vi "f-c_temperature.vi"(10 "Fahrenheit":dbl) -> (2 "Celsius":dbl)   [LabVIEW 2023]
panel:
  out "Thermometer":dbl(slide) scale=0.0..100.0
  out "Numeric 2":dbl
  in  "Numeric":dbl
  out "?":dbl(slide) scale=0.0..100.0
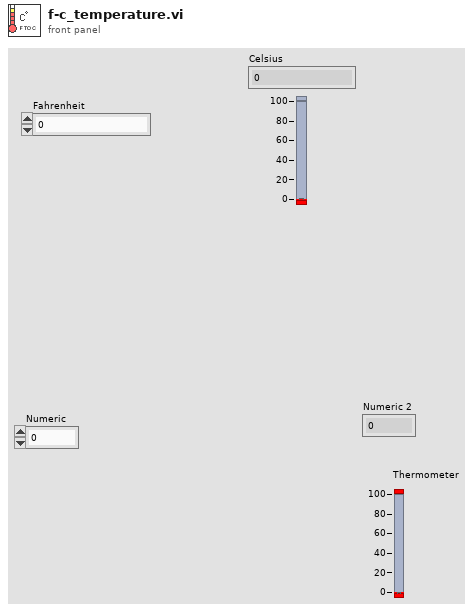
[diagram p1: front panel]
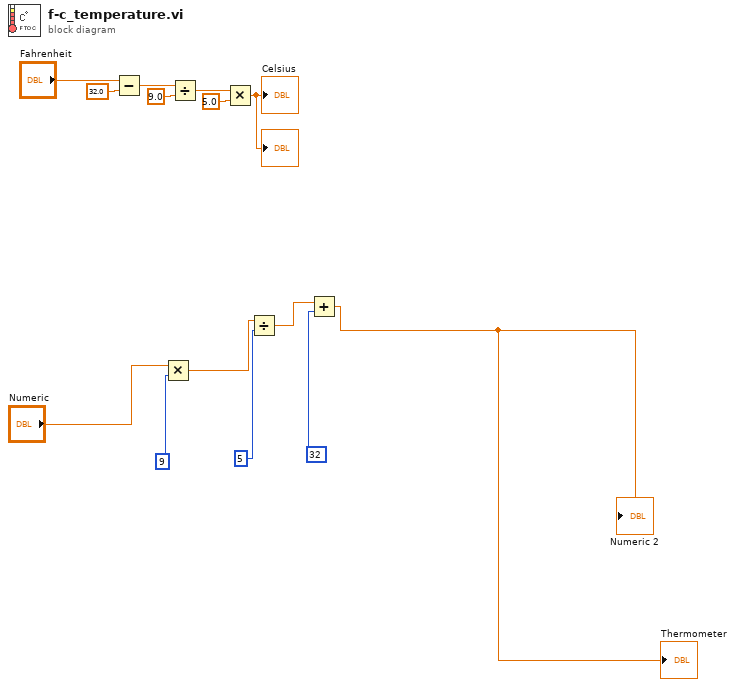
[diagram p0: block diagram]
diagram:
  n1 = Subtract(x="Fahrenheit", y=32.0) -> (x-y=w12:dbl)
  n2 = Multiply(x="Numeric", y=9) -> (x*y=w5:dbl)
  n3 = Divide(x=w12, y=9.0) -> (x/y=w9:dbl)
  n4 = Multiply(x=w9, y=5.0) -> (x*y=→"Celsius" →"?":dbl)
  n5 = Divide(x=w5, y=5) -> (x/y=w3:dbl)
  n6 = Add(x=w3, y=32) -> (x+y=→"Numeric 2" →"Thermometer":dbl)
